vi "GetCustomDeviceRTDriverVIs.vi"(8 "error in (no error)":errorcluster, 11 "custom device reference in":refnum<k39>) -> (0 "error out":errorcluster, 2 "RT driver VIs":T1(array[cluster]), 3 "custom device reference out":refnum<k39>)   [LabVIEW 2027, in "VeriStandTestUtilities.lvlib"]
uses:
  VeriStandTestUtilities.lvlib
  C:/NetCoreDLL/NationalInstruments.VeriStand.XMLReader.dll
  NetCoreDLL/NationalInstruments.VeriStand.XMLReader.dll
  <vilib>/NI VeriStand/Custom Device API/Custom Device Execution Mode.ctl
  <vilib>/NI VeriStand/Custom Device API/Custom Device API.lvlib
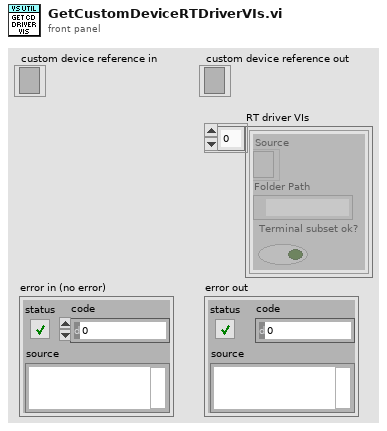
[diagram p1: front panel]
types:
  T1 = cluster{"Source":refnum<k39>, "Folder Path":path, "Terminal subset ok?":bool}[]
  T2 = typedef "Custom Device API.lvlib/Custom Device Execution Mode.ctl" = enum16{"Asynchronous", "Inline HW Interface", "Inline Model Interface", "Inline Timing and Sync", "Asynchronous Timing and Sync"}
  T3 = cluster{"Source":refnum<k39>, "Folder Path":path, bool}
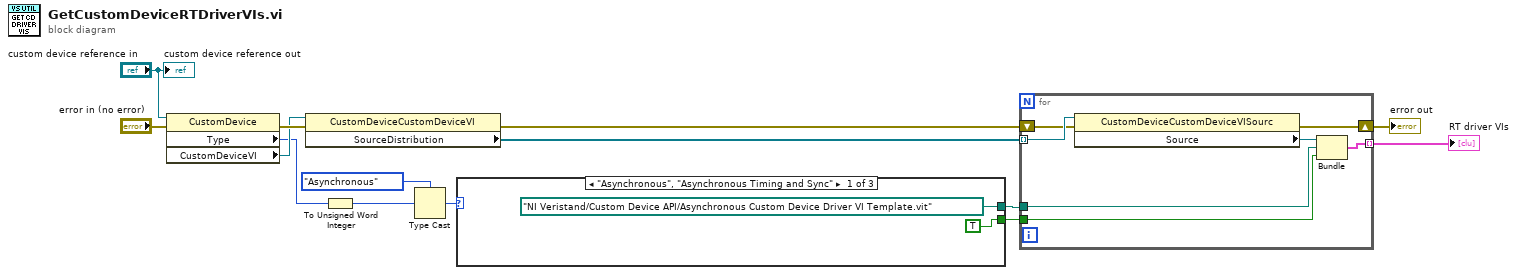
[diagram p0: block diagram]
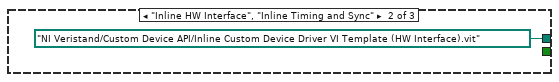
[diagram p2: hidden frame]
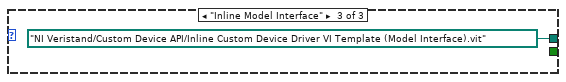
[diagram p3: hidden frame]
diagram:
  n1 = property class="CustomDevice"(reference="custom device reference in", error in="error in (no error)") -> (error out=w14:errorcluster, "Type"=w3:i32, "CustomDeviceVI"=w8:refnum<k39>)  [unwired: 1 out]
  n2 = property class="CustomDeviceCustomDeviceVI"(reference=w8, error in=w14) -> (error out=w11:errorcluster, "SourceDistribution"=w9:refnum<k39>[])  [unwired: 1 out]
  n3 = To Unsigned Word Integer(number=w3) -> (unsigned 16bit integer=w6:u16)
  n4 = Type Cast(type=Custom_Device_Execution_Mode."Asynchronous" ("Execution Mode"), x=w6) -> (*(type *) &x=w4:T2)
  n5 = case shown="\"Asynchronous\", \"Asynchronous Timing and Sync\"" w4 {
    tunnel: [path "NI Veristand/Custom Device API/Asynchronous Custom Device Driver VI Template.vit" ("Folder Path") path "NI Veristand/Custom Device API/Inline Custom Device Driver VI Template (HW Interface).vit" ("Folder Path") path "NI Veristand/Custom Device API/Inline Custom Device Driver VI Template (Model Interface).vit" ("Folder Path")] -> w2
    tunnel: [TRUE _ _] -> w1
    frame "Asynchronous", "Asynchronous Timing and Sync" {
    }
    frame "Inline HW Interface", "Inline Timing and Sync" {
    }
    frame "Inline Model Interface" {
    }
  }
  n6 = for {
    tunnel: w9 -> [w25] mode=indexing
    tunnel: [w23] -> w12 mode=indexing
    shift-right: [w22] -> w10
    shift-left: w11 -> [w21]
    tunnel: w2 -> [w20]
    tunnel: w1 -> [w19]
    n7 = property class="CustomDeviceCustomDeviceVISourc"(reference=w25, error in=w21) -> (error out=w22:errorcluster, "Source"=w24:refnum<k39>)  [unwired: 1 out]
    n8 = Bundle("Source"=w24, "Folder Path"=w20, w19) -> (w23:T3)  [unwired: 1 in]
  }
  "RT driver VIs" <- w12
  "error out" <- w10
  "custom device reference out" <- "custom device reference in"
